vi "Autonomous Independent.vi"   [LabVIEW 2023]
doc: "This VI is called when autonomous begins, and will automatically be terminated when autonomous ends. You can carry out timed or sensor driven robot movement independently without needing to return to the caller."
uses:
  <vilib>/Rock Robotics/WPI/Utilities/WPI_GetSetVariantRefNum.vi
  <vilib>/Rock Robotics/Network Tables/NT Read String.vi
  <vilib>/Rock Robotics/Network Tables/NT Write Numeric Array.vi
  <vilib>/Rock Robotics/WPI/RobotDrive/WPI_RobotDriveMecanumDrive_Cartesian.vi
types:
  T1 = typedef "WPI_JoystickDevRef.ctl" = cluster{"Device":T2}
  T2 = typedef "WPI_JoystickDeviceEnum.ctl" = enum16{"USB 0", "USB 1", "USB 2", "USB 3", "USB 4", "USB 5"}
  T3 = typedef "WPI_RobotDriveDevRef.ctl" = cluster{"DevStatus":errorcluster, "Motors[]":T4[], "Square Inputs":bool, "Max Output":dbl}
  T4 = typedef "WPI_MotorControlDeviceRef.ctl" = cluster{"DeviceStatus":errorcluster, "Type":T5, "PWM":cluster{"PWM Channel":T6, "DeadBand":T7}, "CAN":cluster{"Device Number":u8, "SetOutput VI Ref":variant, "GetOutput VI Ref":variant, "Enable VI Ref":variant, "Disable VI Ref":variant, "Data":variant}, "Invert":bool, "DIO PWM":cluster{"PWM \"Enable\" Channel":T6, "DIOChannel":T8, "PWM Rate":dbl}}
  T5 = typedef "WPI_MotorControlType.ctl" = enum16{"PWM", "CAN", "DIO PWM"}
  T6 = typedef "FPGA_DIOPWMChannel.ctl" = enum8{"PWM 0", "PWM 1", "PWM 2", "PWM 3", "PWM 4", "PWM 5", "PWM 6", "PWM 7", "PWM 8", "PWM 9", "PWM MXP 0", "PWM MXP 1", "PWM MXP 2", "PWM MXP 3", "PWM MXP 4", "PWM MXP 5", "PWM MXP 6", "PWM MXP 7", "PWM MXP 8", "PWM MXP 9", "Invalid"}
  T7 = typedef "WPI_PWMDeadband.ctl" = cluster{"Name":string, "maxPositivePwm":i32, "minPositivePwm":i32, "centerPwm":i32, "maxNegativePwm":i32, "minNegativePwm":i32, "angularRange":u16}
  T8 = typedef "FPGA_DIOChannel.ctl" = enum8{"DIO 0", "DIO 1", "DIO 2", "DIO 3", "DIO 4", "DIO 5", "DIO 6", "DIO 7", "DIO 8", "DIO 9", "DIO MXP 0", "DIO MXP 1", "DIO MXP 2", "DIO MXP 3", "DIO MXP 4", "DIO MXP 5", "DIO MXP 6", "DIO MXP 7", "DIO MXP 8", "DIO MXP 9", "DIO MXP 10", "DIO MXP 11", "DIO MXP 12", "DIO MXP 13", "DIO MXP 14", "DIO MXP 15", "SPI Port CS1", "SPI Port CS2", "SPI Port CS3", "SPI Port MISO", "SPI Port MOSI", "Invalid"}
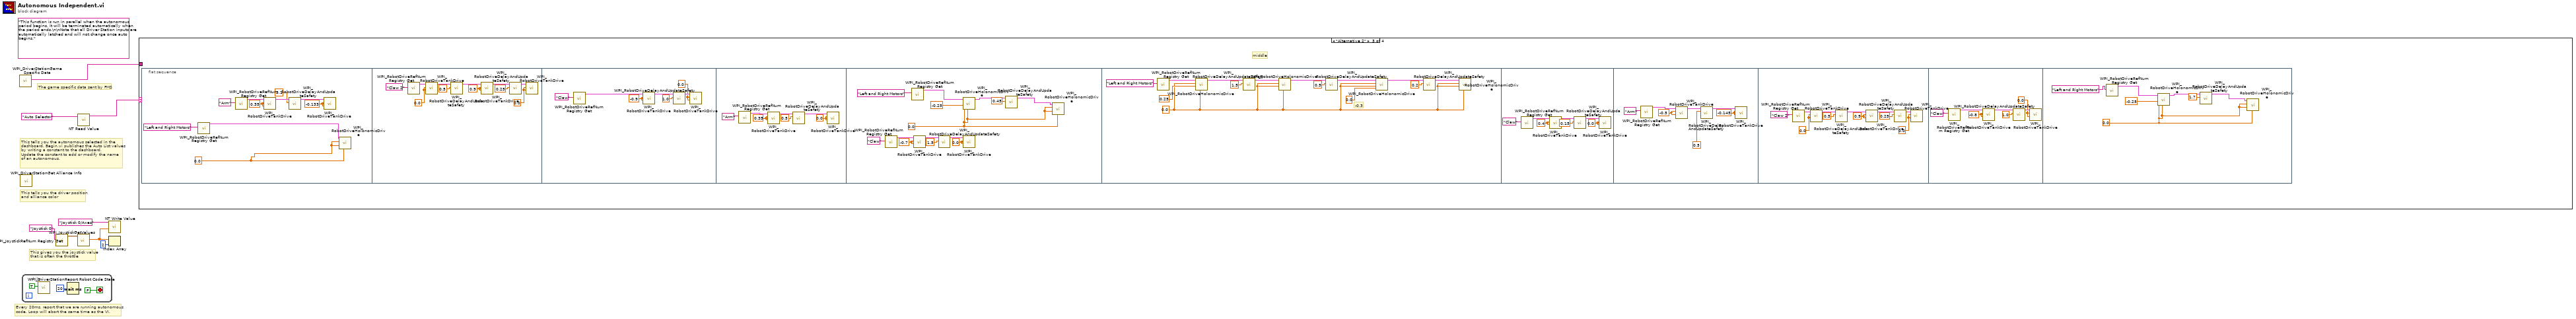
[diagram p0: block diagram]
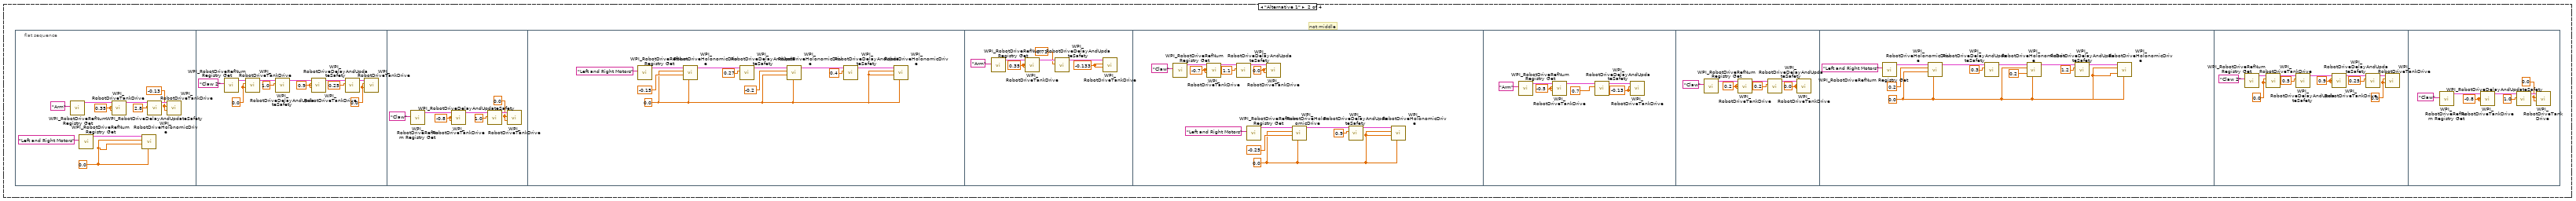
[diagram p3: hidden frame]
diagram:
  (unwired) "This function is run in parallel when the autonomous period begins. It will be terminated automatically when the period ends.\n\nNote that all Driver Station inputs are automatically latched and will not change once auto begins."
  # "The game specific data sent by FMS"
  # "This tells you the autonomous selected in the \ndashboard. Begin.vi publishes the Auto List values\nby writing a constant to the dashboard.\nUpdate the constant to add or modify the name\nof an autonomous."
  # "Every 20ms, report that we are running autonomous\ncode. Loop will abort the same time as the VI."
  # "This gives you the joystick value\nthat is often the throttle"
  # "This tells you the driver position\nand alliance color"
  n1 = call <vilib>:"WPI_DriverStationGame Specific Data.vi"() -> ("Game Specific Data"=w1:string)  [unwired: 11 in]
  n2 = call <vilib>:"WPI_DriverStationGet Alliance Info.vi"() -> ()  [unwired: 12 out]
  n3 = while {
    stop <- FALSE stop-if-true
    n4 = call <vilib>:"WPI_DriverStationReport Robot Code State.vi"("Autonomous"=TRUE) -> ()  [unwired: 10 in, 1 out]
    n5 = Wait (ms)(milliseconds to wait=u32 20) -> ()  [unwired: 1 out]
  }
  n6 = call <vilib>:"WPI_JoystickRefNum Registry Get.vi"("refnum name"="Joystick 0") -> ("JoystickDevRef"=w7:T1)  [unwired: 1 in, 9 out]
  n7 = call <vilib>:"WPI_JoystickGetValues.vi"("JoystickDevRef"=w7) -> ("Axes"=w3:dbl[])  [unwired: 6 in, 4 out]
  n8 = call-poly <vilib>:"NT Read Value.vi"("name"="Auto Selector" ("Name")) -> ("value"=w4:string)  [unwired: 8 in, 2 out]
  n9 = call-poly <vilib>:"NT Write Value.vi"("value"=w3, "name"="Joystick 0/Axes" ("Name")) -> ()  [unwired: 9 in, 1 out]
  n10 = Index Array(array=w3, index=2) -> ()  [unwired: 1 out]
  n11 = case shown="\"Alternative 2\"" w4 {
    tunnel: w1 -> [_ _ _ _]
    frame Default {
      # "You can put your main auto here, or you can right-click on the case and make any\nother frame be the default case."
      # "This is the frame that will execute if no selection is made, or if it is not recognized"
    }
    frame "Alternative 1" {
      # "not middle"
      n12 = flat-sequence {
        frame #0 {
          w12 = 0.0
          w16 = 0.35 ("Left axis value")
          w18 = -0.13 ("Left axis value")
          n13 = call <vilib>:"WPI_RobotDriveRefNum Registry Get.vi"("refnum name"="Arm") -> ("RobotDriveDevRef"=w21:T3)  [unwired: 1 in, 9 out]
          n14 = call <vilib>:"WPI_RobotDriveRefNum Registry Get.vi"("refnum name"="Left and Right Motors") -> ("RobotDriveDevRef"=w14:T3)  [unwired: 1 in, 9 out]
          n15 = call <vilib>:"WPI_RobotDriveTankDrive.vi"("Right axis value"=w16, "Left axis value"=w16, "RobotDriveDevRef"=w21) -> ("RobotDriveDevRef"=w19:T3)  [unwired: 6 in, 2 out]
          n16 = call-poly <vilib>:"WPI_RobotDriveHolonomicDrive.vi"("Rotation"=w12, "Y"=w12, "X"=w12, "RobotDriveDevRef"=w14) -> ()  [unwired: 5 in, 3 out]
          n17 = call <vilib>:"WPI_RobotDriveDelayAndUpdateSafety.vi"("Delay (s)"=2.8, "RobotDriveDevRef"=w19) -> ("RobotDriveDevRef 2"=w20:T3)  [unwired: 8 in, 1 out]
          n18 = call <vilib>:"WPI_RobotDriveTankDrive.vi"("Right axis value"=w18, "Left axis value"=w18, "RobotDriveDevRef"=w20) -> ()  [unwired: 6 in, 3 out]
        }
        frame #1 {
          w27 = 0.0 ("Left axis value")
          w26 = 0.0 ("Left axis value")
          w23 = 0.9 ("Left axis value")
          n19 = call <vilib>:"WPI_RobotDriveRefNum Registry Get.vi"("refnum name"="Claw 2") -> ("RobotDriveDevRef"=w32:T3)  [unwired: 1 in, 9 out]
          n20 = call <vilib>:"WPI_RobotDriveTankDrive.vi"("Right axis value"=w27, "Left axis value"=w27, "RobotDriveDevRef"=w32) -> ("RobotDriveDevRef"=w31:T3)  [unwired: 6 in, 2 out]
          n21 = call <vilib>:"WPI_RobotDriveDelayAndUpdateSafety.vi"("Delay (s)"=1.0, "RobotDriveDevRef"=w31) -> ("RobotDriveDevRef 2"=w28:T3)  [unwired: 8 in, 1 out]
          n22 = call <vilib>:"WPI_RobotDriveTankDrive.vi"("Right axis value"=w23, "Left axis value"=w23, "RobotDriveDevRef"=w28) -> ("RobotDriveDevRef"=w30:T3)  [unwired: 6 in, 2 out]
          n23 = call <vilib>:"WPI_RobotDriveDelayAndUpdateSafety.vi"("Delay (s)"=0.25, "RobotDriveDevRef"=w30) -> ("RobotDriveDevRef 2"=w29:T3)  [unwired: 8 in, 1 out]
          n24 = call <vilib>:"WPI_RobotDriveTankDrive.vi"("Right axis value"=w26, "Left axis value"=w26, "RobotDriveDevRef"=w29) -> ()  [unwired: 6 in, 3 out]
        }
        frame #2 {
          w34 = -0.8 ("Left axis value")
          w36 = 0.0 ("Left axis value")
          n25 = call <vilib>:"WPI_RobotDriveRefNum Registry Get.vi"("refnum name"="Claw") -> ("RobotDriveDevRef"=w39:T3)  [unwired: 1 in, 9 out]
          n26 = call <vilib>:"WPI_RobotDriveTankDrive.vi"("Right axis value"=w34, "Left axis value"=w34, "RobotDriveDevRef"=w39) -> ("RobotDriveDevRef"=w37:T3)  [unwired: 6 in, 2 out]
          n27 = call <vilib>:"WPI_RobotDriveDelayAndUpdateSafety.vi"("Delay (s)"=1.0, "RobotDriveDevRef"=w37) -> ("RobotDriveDevRef 2"=w38:T3)  [unwired: 8 in, 1 out]
          n28 = call <vilib>:"WPI_RobotDriveTankDrive.vi"("Right axis value"=w36, "Left axis value"=w36, "RobotDriveDevRef"=w38) -> ()  [unwired: 6 in, 3 out]
        }
        frame #3 {
          w40 = 0.0 ("X")
          n29 = call <vilib>:"WPI_RobotDriveRefNum Registry Get.vi"("refnum name"="Left and Right Motors") -> ("RobotDriveDevRef"=w50:T3)  [unwired: 1 in, 9 out]
          n30 = call-poly <vilib>:"WPI_RobotDriveHolonomicDrive.vi"("Rotation"=w40, "Y"=-0.15 ("X"), "X"=w40, "RobotDriveDevRef"=w50) -> ("RobotDriveDevRef"=w49:T3)  [unwired: 5 in, 2 out]
          n31 = call <vilib>:"WPI_RobotDriveDelayAndUpdateSafety.vi"("Delay (s)"=0.27, "RobotDriveDevRef"=w49) -> ("RobotDriveDevRef 2"=w48:T3)  [unwired: 8 in, 1 out]
          n32 = call-poly <vilib>:"WPI_RobotDriveHolonomicDrive.vi"("Rotation"=w40, "Y"=w40, "X"=-0.2, "RobotDriveDevRef"=w48) -> ("RobotDriveDevRef"=w46:T3)  [unwired: 5 in, 2 out]
          n33 = call <vilib>:"WPI_RobotDriveDelayAndUpdateSafety.vi"("Delay (s)"=0.4, "RobotDriveDevRef"=w46) -> ("RobotDriveDevRef 2"=w44:T3)  [unwired: 8 in, 1 out]
          n34 = call-poly <vilib>:"WPI_RobotDriveHolonomicDrive.vi"("Rotation"=w40, "Y"=w40, "X"=w40, "RobotDriveDevRef"=w44) -> ()  [unwired: 5 in, 3 out]
        }
        frame #4 {
          w54 = -0.133 ("Left axis value")
          w53 = 0.35 ("t")
          n35 = call <vilib>:"WPI_RobotDriveRefNum Registry Get.vi"("refnum name"="Arm") -> ("RobotDriveDevRef"=w55:T3)  [unwired: 1 in, 9 out]
          n36 = call <vilib>:"WPI_RobotDriveTankDrive.vi"("Right axis value"=w53, "Left axis value"=w53, "RobotDriveDevRef"=w55) -> ("RobotDriveDevRef"=w56:T3)  [unwired: 6 in, 2 out]
          n37 = call <vilib>:"WPI_RobotDriveDelayAndUpdateSafety.vi"("Delay (s)"=0.71, "RobotDriveDevRef"=w56) -> ("RobotDriveDevRef 2"=w57:T3)  [unwired: 8 in, 1 out]
          n38 = call <vilib>:"WPI_RobotDriveTankDrive.vi"("Right axis value"=w54, "Left axis value"=w54, "RobotDriveDevRef"=w57) -> ()  [unwired: 6 in, 3 out]
        }
        frame #5 {
          w58 = 0.0 ("X")
          w67 = 0.0 ("Left axis value")
          w65 = -0.7 ("Left axis value")
          n39 = call <vilib>:"WPI_RobotDriveRefNum Registry Get.vi"("refnum name"="Claw") -> ("RobotDriveDevRef"=w70:T3)  [unwired: 1 in, 9 out]
          n40 = call <vilib>:"WPI_RobotDriveTankDrive.vi"("Right axis value"=w65, "Left axis value"=w65, "RobotDriveDevRef"=w70) -> ("RobotDriveDevRef"=w71:T3)  [unwired: 6 in, 2 out]
          n41 = call <vilib>:"WPI_RobotDriveDelayAndUpdateSafety.vi"("Delay (s)"=1.1, "RobotDriveDevRef"=w71) -> ("RobotDriveDevRef 2"=w69:T3)  [unwired: 8 in, 1 out]
          n42 = call <vilib>:"WPI_RobotDriveRefNum Registry Get.vi"("refnum name"="Left and Right Motors") -> ("RobotDriveDevRef"=w59:T3)  [unwired: 1 in, 9 out]
          n43 = call <vilib>:"WPI_RobotDriveTankDrive.vi"("Right axis value"=w67, "Left axis value"=w67, "RobotDriveDevRef"=w69) -> ()  [unwired: 6 in, 3 out]
          n44 = call-poly <vilib>:"WPI_RobotDriveHolonomicDrive.vi"("Rotation"=w58, "Y"=-0.25 ("X"), "X"=w58, "RobotDriveDevRef"=w59) -> ("RobotDriveDevRef"=w63:T3)  [unwired: 5 in, 2 out]
          n45 = call <vilib>:"WPI_RobotDriveDelayAndUpdateSafety.vi"("Delay (s)"=0.9, "RobotDriveDevRef"=w63) -> ("RobotDriveDevRef 2"=w64:T3)  [unwired: 8 in, 1 out]
          n46 = call-poly <vilib>:"WPI_RobotDriveHolonomicDrive.vi"("Rotation"=w58, "Y"=w58, "X"=w58, "RobotDriveDevRef"=w64) -> ()  [unwired: 5 in, 3 out]
        }
        frame #6 {
          w75 = -0.13 ("Left axis value")
          w74 = -0.5 ("t")
          n47 = call <vilib>:"WPI_RobotDriveRefNum Registry Get.vi"("refnum name"="Arm") -> ("RobotDriveDevRef"=w78:T3)  [unwired: 1 in, 9 out]
          n48 = call <vilib>:"WPI_RobotDriveTankDrive.vi"("Right axis value"=w74, "Left axis value"=w74, "RobotDriveDevRef"=w78) -> ("RobotDriveDevRef"=w77:T3)  [unwired: 6 in, 2 out]
          n49 = call <vilib>:"WPI_RobotDriveDelayAndUpdateSafety.vi"("Delay (s)"=0.7, "RobotDriveDevRef"=w77) -> ("RobotDriveDevRef 2"=w76:T3)  [unwired: 8 in, 1 out]
          n50 = call <vilib>:"WPI_RobotDriveTankDrive.vi"("Right axis value"=w75, "Left axis value"=w75, "RobotDriveDevRef"=w76) -> ()  [unwired: 6 in, 3 out]
        }
        frame #7 {
          w81 = 0.0 ("Left axis value")
          w79 = 0.2 ("Left axis value")
          n51 = call <vilib>:"WPI_RobotDriveRefNum Registry Get.vi"("refnum name"="Claw") -> ("RobotDriveDevRef"=w84:T3)  [unwired: 1 in, 9 out]
          n52 = call <vilib>:"WPI_RobotDriveTankDrive.vi"("Right axis value"=w79, "Left axis value"=w79, "RobotDriveDevRef"=w84) -> ("RobotDriveDevRef"=w83:T3)  [unwired: 6 in, 2 out]
          n53 = call <vilib>:"WPI_RobotDriveDelayAndUpdateSafety.vi"("Delay (s)"=0.2, "RobotDriveDevRef"=w83) -> ("RobotDriveDevRef 2"=w85:T3)  [unwired: 8 in, 1 out]
          n54 = call <vilib>:"WPI_RobotDriveTankDrive.vi"("Right axis value"=w81, "Left axis value"=w81, "RobotDriveDevRef"=w85) -> ()  [unwired: 6 in, 3 out]
        }
        frame #8 {
          w86 = 0.0 ("X")
          n55 = call <vilib>:"WPI_RobotDriveRefNum Registry Get.vi"("refnum name"="Left and Right Motors") -> ("RobotDriveDevRef"=w96:T3)  [unwired: 1 in, 9 out]
          n56 = call-poly <vilib>:"WPI_RobotDriveHolonomicDrive.vi"("Rotation"=w86, "Y"=w86, "X"=0.2, "RobotDriveDevRef"=w96) -> ("RobotDriveDevRef"=w95:T3)  [unwired: 5 in, 2 out]
          n57 = call <vilib>:"WPI_RobotDriveDelayAndUpdateSafety.vi"("Delay (s)"=0.3, "RobotDriveDevRef"=w95) -> ("RobotDriveDevRef 2"=w94:T3)  [unwired: 8 in, 1 out]
          n58 = call-poly <vilib>:"WPI_RobotDriveHolonomicDrive.vi"("Rotation"=w86, "Y"=0.2, "X"=w86, "RobotDriveDevRef"=w94) -> ("RobotDriveDevRef"=w87:T3)  [unwired: 5 in, 2 out]
          n59 = call <vilib>:"WPI_RobotDriveDelayAndUpdateSafety.vi"("Delay (s)"=1.2, "RobotDriveDevRef"=w87) -> ("RobotDriveDevRef 2"=w89:T3)  [unwired: 8 in, 1 out]
          n60 = call-poly <vilib>:"WPI_RobotDriveHolonomicDrive.vi"("Rotation"=w86, "Y"=w86, "X"=w86, "RobotDriveDevRef"=w89) -> ()  [unwired: 5 in, 3 out]
        }
        frame #9 {
          w102 = 0.0 ("Left axis value")
          w101 = 0.0 ("Left axis value")
          w98 = 0.9 ("Left axis value")
          n61 = call <vilib>:"WPI_RobotDriveRefNum Registry Get.vi"("refnum name"="Claw 2") -> ("RobotDriveDevRef"=w103:T3)  [unwired: 1 in, 9 out]
          n62 = call <vilib>:"WPI_RobotDriveTankDrive.vi"("Right axis value"=w102, "Left axis value"=w102, "RobotDriveDevRef"=w103) -> ("RobotDriveDevRef"=w104:T3)  [unwired: 6 in, 2 out]
          n63 = call <vilib>:"WPI_RobotDriveDelayAndUpdateSafety.vi"("Delay (s)"=0.5, "RobotDriveDevRef"=w104) -> ("RobotDriveDevRef 2"=w107:T3)  [unwired: 8 in, 1 out]
          n64 = call <vilib>:"WPI_RobotDriveTankDrive.vi"("Right axis value"=w98, "Left axis value"=w98, "RobotDriveDevRef"=w107) -> ("RobotDriveDevRef"=w105:T3)  [unwired: 6 in, 2 out]
          n65 = call <vilib>:"WPI_RobotDriveDelayAndUpdateSafety.vi"("Delay (s)"=0.25, "RobotDriveDevRef"=w105) -> ("RobotDriveDevRef 2"=w106:T3)  [unwired: 8 in, 1 out]
          n66 = call <vilib>:"WPI_RobotDriveTankDrive.vi"("Right axis value"=w101, "Left axis value"=w101, "RobotDriveDevRef"=w106) -> ()  [unwired: 6 in, 3 out]
        }
        frame #10 {
          w109 = -0.8 ("Left axis value")
          w111 = 0.0 ("Left axis value")
          n67 = call <vilib>:"WPI_RobotDriveRefNum Registry Get.vi"("refnum name"="Claw") -> ("RobotDriveDevRef"=w112:T3)  [unwired: 1 in, 9 out]
          n68 = call <vilib>:"WPI_RobotDriveTankDrive.vi"("Right axis value"=w109, "Left axis value"=w109, "RobotDriveDevRef"=w112) -> ("RobotDriveDevRef"=w114:T3)  [unwired: 6 in, 2 out]
          n69 = call <vilib>:"WPI_RobotDriveDelayAndUpdateSafety.vi"("Delay (s)"=1.0, "RobotDriveDevRef"=w114) -> ("RobotDriveDevRef 2"=w113:T3)  [unwired: 8 in, 1 out]
          n70 = call <vilib>:"WPI_RobotDriveTankDrive.vi"("Right axis value"=w111, "Left axis value"=w111, "RobotDriveDevRef"=w113) -> ()  [unwired: 6 in, 3 out]
        }
      }
    }
    frame "Alternative 2" {
      # "middle"
      n71 = flat-sequence {
        frame #0 {
          w116 = 0.0 ("X")
          w121 = -0.133 ("Left axis value")
          w120 = 0.35 ("t")
          n72 = call <vilib>:"WPI_RobotDriveRefNum Registry Get.vi"("refnum name"="Left and Right Motors") -> ("RobotDriveDevRef"=w115:T3)  [unwired: 1 in, 9 out]
          n73 = call <vilib>:"WPI_RobotDriveRefNum Registry Get.vi"("refnum name"="Arm") -> ("RobotDriveDevRef"=w122:T3)  [unwired: 1 in, 9 out]
          n74 = call <vilib>:"WPI_RobotDriveTankDrive.vi"("Right axis value"=w120, "Left axis value"=w120, "RobotDriveDevRef"=w122) -> ("RobotDriveDevRef"=w123:T3)  [unwired: 6 in, 2 out]
          n75 = call <vilib>:"WPI_RobotDriveDelayAndUpdateSafety.vi"("Delay (s)"=3.1, "RobotDriveDevRef"=w123) -> ("RobotDriveDevRef 2"=w124:T3)  [unwired: 8 in, 1 out]
          n76 = call <vilib>:"WPI_RobotDriveTankDrive.vi"("Right axis value"=w121, "Left axis value"=w121, "RobotDriveDevRef"=w124) -> ()  [unwired: 6 in, 3 out]
          n77 = call-poly <vilib>:"WPI_RobotDriveHolonomicDrive.vi"("Rotation"=w116, "Y"=w116, "X"=w116, "RobotDriveDevRef"=w115) -> ()  [unwired: 5 in, 3 out]
        }
        frame #1 {
          w135 = 0.0 ("Left axis value")
          w134 = 0.0 ("Left axis value")
          w125 = 0.9 ("Left axis value")
          n78 = call <vilib>:"WPI_RobotDriveRefNum Registry Get.vi"("refnum name"="Claw 2") -> ("RobotDriveDevRef"=w130:T3)  [unwired: 1 in, 9 out]
          n79 = call <vilib>:"WPI_RobotDriveTankDrive.vi"("Right axis value"=w135, "Left axis value"=w135, "RobotDriveDevRef"=w130) -> ("RobotDriveDevRef"=w129:T3)  [unwired: 6 in, 2 out]
          n80 = call <vilib>:"WPI_RobotDriveDelayAndUpdateSafety.vi"("Delay (s)"=0.5, "RobotDriveDevRef"=w129) -> ("RobotDriveDevRef 2"=w126:T3)  [unwired: 8 in, 1 out]
          n81 = call <vilib>:"WPI_RobotDriveTankDrive.vi"("Right axis value"=w125, "Left axis value"=w125, "RobotDriveDevRef"=w126) -> ("RobotDriveDevRef"=w128:T3)  [unwired: 6 in, 2 out]
          n82 = call <vilib>:"WPI_RobotDriveDelayAndUpdateSafety.vi"("Delay (s)"=0.25, "RobotDriveDevRef"=w128) -> ("RobotDriveDevRef 2"=w127:T3)  [unwired: 8 in, 1 out]
          n83 = call <vilib>:"WPI_RobotDriveTankDrive.vi"("Right axis value"=w134, "Left axis value"=w134, "RobotDriveDevRef"=w127) -> ()  [unwired: 6 in, 3 out]
        }
        frame #2 {
          w139 = -0.9 ("Left axis value")
          w137 = 0.0 ("Left axis value")
          n84 = call <vilib>:"WPI_RobotDriveRefNum Registry Get.vi"("refnum name"="Claw") -> ("RobotDriveDevRef"=w136:T3)  [unwired: 1 in, 9 out]
          n85 = call <vilib>:"WPI_RobotDriveTankDrive.vi"("Right axis value"=w139, "Left axis value"=w139, "RobotDriveDevRef"=w136) -> ("RobotDriveDevRef"=w142:T3)  [unwired: 6 in, 2 out]
          n86 = call <vilib>:"WPI_RobotDriveDelayAndUpdateSafety.vi"("Delay (s)"=1.0, "RobotDriveDevRef"=w142) -> ("RobotDriveDevRef 2"=w141:T3)  [unwired: 8 in, 1 out]
          n87 = call <vilib>:"WPI_RobotDriveTankDrive.vi"("Right axis value"=w137, "Left axis value"=w137, "RobotDriveDevRef"=w141) -> ()  [unwired: 6 in, 3 out]
        }
        frame #3 {
          w146 = 0.0 ("Left axis value")
          w145 = 0.35 ("t")
          n88 = call <vilib>:"WPI_RobotDriveRefNum Registry Get.vi"("refnum name"="Arm") -> ("RobotDriveDevRef"=w147:T3)  [unwired: 1 in, 9 out]
          n89 = call <vilib>:"WPI_RobotDriveTankDrive.vi"("Right axis value"=w145, "Left axis value"=w145, "RobotDriveDevRef"=w147) -> ("RobotDriveDevRef"=w148:T3)  [unwired: 6 in, 2 out]
          n90 = call <vilib>:"WPI_RobotDriveDelayAndUpdateSafety.vi"("Delay (s)"=0.5, "RobotDriveDevRef"=w148) -> ("RobotDriveDevRef 2"=w149:T3)  [unwired: 8 in, 1 out]
          n91 = call <vilib>:"WPI_RobotDriveTankDrive.vi"("Right axis value"=w146, "Left axis value"=w146, "RobotDriveDevRef"=w149) -> ()  [unwired: 6 in, 3 out]
        }
        frame #4 {
          w152 = 0.0 ("Left axis value")
          w150 = -0.7 ("Left axis value")
          w157 = 0.0 ("X")
          n92 = call <vilib>:"WPI_RobotDriveRefNum Registry Get.vi"("refnum name"="Claw") -> ("RobotDriveDevRef"=w155:T3)  [unwired: 1 in, 9 out]
          n93 = call <vilib>:"WPI_RobotDriveRefNum Registry Get.vi"("refnum name"="Left and Right Motors") -> ("RobotDriveDevRef"=w162:T3)  [unwired: 1 in, 9 out]
          n94 = call <vilib>:"WPI_RobotDriveTankDrive.vi"("Right axis value"=w150, "Left axis value"=w150, "RobotDriveDevRef"=w155) -> ("RobotDriveDevRef"=w156:T3)  [unwired: 6 in, 2 out]
          n95 = call <vilib>:"WPI_RobotDriveDelayAndUpdateSafety.vi"("Delay (s)"=1.5, "RobotDriveDevRef"=w156) -> ("RobotDriveDevRef 2"=w154:T3)  [unwired: 8 in, 1 out]
          n96 = call-poly <vilib>:"WPI_RobotDriveHolonomicDrive.vi"("Rotation"=w157, "Y"=-0.25, "X"=w157, "RobotDriveDevRef"=w162) -> ("RobotDriveDevRef"=w160:T3)  [unwired: 5 in, 2 out]
          n97 = call <vilib>:"WPI_RobotDriveTankDrive.vi"("Right axis value"=w152, "Left axis value"=w152, "RobotDriveDevRef"=w154) -> ()  [unwired: 6 in, 3 out]
          n98 = call <vilib>:"WPI_RobotDriveDelayAndUpdateSafety.vi"("Delay (s)"=0.45, "RobotDriveDevRef"=w160) -> ("RobotDriveDevRef 2"=w158:T3)  [unwired: 8 in, 1 out]
          n99 = call-poly <vilib>:"WPI_RobotDriveHolonomicDrive.vi"("Rotation"=w157, "Y"=w157, "X"=w157, "RobotDriveDevRef"=w158) -> ()  [unwired: 5 in, 3 out]
        }
        frame #5 {
          w168 = 0.0 ("X")
          # "-0.3"
          n100 = call <vilib>:"WPI_RobotDriveRefNum Registry Get.vi"("refnum name"="Left and Right Motors") -> ("RobotDriveDevRef"=w177:T3)  [unwired: 1 in, 9 out]
          n101 = call-poly <vilib>:"WPI_RobotDriveHolonomicDrive.vi"("Rotation"=w168, "Y"=0.25, "X"=w168, "RobotDriveDevRef"=w177) -> ("RobotDriveDevRef"=w175:T3)  [unwired: 5 in, 2 out]
          n102 = call <vilib>:"WPI_RobotDriveDelayAndUpdateSafety.vi"("Delay (s)"=1.5, "RobotDriveDevRef"=w175) -> ("RobotDriveDevRef 2"=w167:T3)  [unwired: 8 in, 1 out]
          n103 = call-poly <vilib>:"WPI_RobotDriveHolonomicDrive.vi"("Rotation"=w168, "Y"=w168, "X"=w168, "RobotDriveDevRef"=w167) -> ("RobotDriveDevRef"=w165:T3)  [unwired: 5 in, 2 out]
          n104 = call <vilib>:"WPI_RobotDriveDelayAndUpdateSafety.vi"("Delay (s)"=0.5, "RobotDriveDevRef"=w165) -> ("RobotDriveDevRef 2"=w164:T3)  [unwired: 8 in, 1 out]
          n105 = call-poly <vilib>:"WPI_RobotDriveHolonomicDrive.vi"("Rotation"=0.0, "Y"=w168, "X"=w168, "RobotDriveDevRef"=w164) -> ("RobotDriveDevRef"=w171:T3)  [unwired: 5 in, 2 out]
          n106 = call <vilib>:"WPI_RobotDriveDelayAndUpdateSafety.vi"("Delay (s)"=0.2, "RobotDriveDevRef"=w171) -> ("RobotDriveDevRef 2"=w170:T3)  [unwired: 8 in, 1 out]
          n107 = call-poly <vilib>:"WPI_RobotDriveHolonomicDrive.vi"("Rotation"=w168, "Y"=w168, "X"=w168, "RobotDriveDevRef"=w170) -> ()  [unwired: 5 in, 3 out]
        }
        frame #6 {
          w180 = 0.0 ("Left axis value")
          w178 = 0.4 ("Left axis value")
          n108 = call <vilib>:"WPI_RobotDriveRefNum Registry Get.vi"("refnum name"="Claw") -> ("RobotDriveDevRef"=w183:T3)  [unwired: 1 in, 9 out]
          n109 = call <vilib>:"WPI_RobotDriveTankDrive.vi"("Right axis value"=w178, "Left axis value"=w178, "RobotDriveDevRef"=w183) -> ("RobotDriveDevRef"=w184:T3)  [unwired: 6 in, 2 out]
          n110 = call <vilib>:"WPI_RobotDriveDelayAndUpdateSafety.vi"("Delay (s)"=0.15, "RobotDriveDevRef"=w184) -> ("RobotDriveDevRef 2"=w182:T3)  [unwired: 8 in, 1 out]
          n111 = call <vilib>:"WPI_RobotDriveTankDrive.vi"("Right axis value"=w180, "Left axis value"=w180, "RobotDriveDevRef"=w182) -> ()  [unwired: 6 in, 3 out]
        }
        frame #7 {
          w188 = -0.145 ("Left axis value")
          w187 = -0.5 ("t")
          n112 = call <vilib>:"WPI_RobotDriveRefNum Registry Get.vi"("refnum name"="Arm") -> ("RobotDriveDevRef"=w189:T3)  [unwired: 1 in, 9 out]
          n113 = call <vilib>:"WPI_RobotDriveTankDrive.vi"("Right axis value"=w187, "Left axis value"=w187, "RobotDriveDevRef"=w189) -> ("RobotDriveDevRef"=w190:T3)  [unwired: 6 in, 2 out]
          n114 = call <vilib>:"WPI_RobotDriveDelayAndUpdateSafety.vi"("Delay (s)"=0.5, "RobotDriveDevRef"=w190) -> ("RobotDriveDevRef 2"=w191:T3)  [unwired: 8 in, 1 out]
          n115 = call <vilib>:"WPI_RobotDriveTankDrive.vi"("Right axis value"=w188, "Left axis value"=w188, "RobotDriveDevRef"=w191) -> ()  [unwired: 6 in, 3 out]
        }
        frame #8 {
          w202 = 0.0 ("Left axis value")
          w201 = 0.0 ("Left axis value")
          w192 = 0.9 ("Left axis value")
          n116 = call <vilib>:"WPI_RobotDriveRefNum Registry Get.vi"("refnum name"="Claw 2") -> ("RobotDriveDevRef"=w197:T3)  [unwired: 1 in, 9 out]
          n117 = call <vilib>:"WPI_RobotDriveTankDrive.vi"("Right axis value"=w202, "Left axis value"=w202, "RobotDriveDevRef"=w197) -> ("RobotDriveDevRef"=w196:T3)  [unwired: 6 in, 2 out]
          n118 = call <vilib>:"WPI_RobotDriveDelayAndUpdateSafety.vi"("Delay (s)"=0.5, "RobotDriveDevRef"=w196) -> ("RobotDriveDevRef 2"=w193:T3)  [unwired: 8 in, 1 out]
          n119 = call <vilib>:"WPI_RobotDriveTankDrive.vi"("Right axis value"=w192, "Left axis value"=w192, "RobotDriveDevRef"=w193) -> ("RobotDriveDevRef"=w195:T3)  [unwired: 6 in, 2 out]
          n120 = call <vilib>:"WPI_RobotDriveDelayAndUpdateSafety.vi"("Delay (s)"=0.25, "RobotDriveDevRef"=w195) -> ("RobotDriveDevRef 2"=w194:T3)  [unwired: 8 in, 1 out]
          n121 = call <vilib>:"WPI_RobotDriveTankDrive.vi"("Right axis value"=w201, "Left axis value"=w201, "RobotDriveDevRef"=w194) -> ()  [unwired: 6 in, 3 out]
        }
        frame #9 {
          w204 = -0.8 ("Left axis value")
          w206 = 0.0 ("Left axis value")
          n122 = call <vilib>:"WPI_RobotDriveRefNum Registry Get.vi"("refnum name"="Claw") -> ("RobotDriveDevRef"=w209:T3)  [unwired: 1 in, 9 out]
          n123 = call <vilib>:"WPI_RobotDriveTankDrive.vi"("Right axis value"=w204, "Left axis value"=w204, "RobotDriveDevRef"=w209) -> ("RobotDriveDevRef"=w207:T3)  [unwired: 6 in, 2 out]
          n124 = call <vilib>:"WPI_RobotDriveDelayAndUpdateSafety.vi"("Delay (s)"=1.0, "RobotDriveDevRef"=w207) -> ("RobotDriveDevRef 2"=w208:T3)  [unwired: 8 in, 1 out]
          n125 = call <vilib>:"WPI_RobotDriveTankDrive.vi"("Right axis value"=w206, "Left axis value"=w206, "RobotDriveDevRef"=w208) -> ()  [unwired: 6 in, 3 out]
        }
        frame #10 {
          w211 = 0.0 ("X")
          n126 = call <vilib>:"WPI_RobotDriveRefNum Registry Get.vi"("refnum name"="Left and Right Motors") -> ("RobotDriveDevRef"=w216:T3)  [unwired: 1 in, 9 out]
          n127 = call-poly <vilib>:"WPI_RobotDriveHolonomicDrive.vi"("Rotation"=w211, "Y"=-0.25, "X"=w211, "RobotDriveDevRef"=w216) -> ("RobotDriveDevRef"=w214:T3)  [unwired: 5 in, 2 out]
          n128 = call <vilib>:"WPI_RobotDriveDelayAndUpdateSafety.vi"("Delay (s)"=1.7, "RobotDriveDevRef"=w214) -> ("RobotDriveDevRef 2"=w212:T3)  [unwired: 8 in, 1 out]
          n129 = call-poly <vilib>:"WPI_RobotDriveHolonomicDrive.vi"("Rotation"=w211, "Y"=w211, "X"=w211, "RobotDriveDevRef"=w212) -> ()  [unwired: 5 in, 3 out]
        }
      }
    }
    frame "Your Turn" {
    }
  }
